vi "Send Text Using SMTP API 2013 NIVerified.vi"(2 "phone number 2":string, 3 "Carrier 2":enum16{"T-Mobile", "AT&T", "Verizon", "Sprint"}(ring), 4 "Body":string, 5 "Carrier 1":enum16{"T-Mobile", "AT&T", "Verizon", "Sprint"}(ring), 6 "Subject":string, 7 "phone number 1":string, 9 "Outgoing Mail Server (SMTP)":string="smtp.gmail.com", 10 "Password":string, 11 "Email":string) -> ()   [LabVIEW 2018]
uses:
  <vilib>/smtpClient/Set Message Text.vi
  <vilib>/smtpClient/LabVIEWSMTPClient.lvlib
panel:
  in  "TLS":bool=TRUE
  # "Overview\nThis example will allows you to use an SMTP server to send a SMS message to a cell phone.\nDescription\nWith the SMTP API you can send an email to your phone as a text message.  There are a lot of different servers you\n can use the default in this example is using GMAIL through the smtp.gmail.com server.  Most SMTP servers should \nwork, but the server and cell phone needs to be compatible to send and receive SMS messages.\nSteps to Implement or Execute Code\nOpen Send Text using SMTP API.vi\nFill in the SMTP server in the Outgoing Mail Server (SMTP), gmail is the default server\nFill out your email & Password\nSelect your Carrier and Type your Phone Number\nType the text you would like to send in the Body Control"
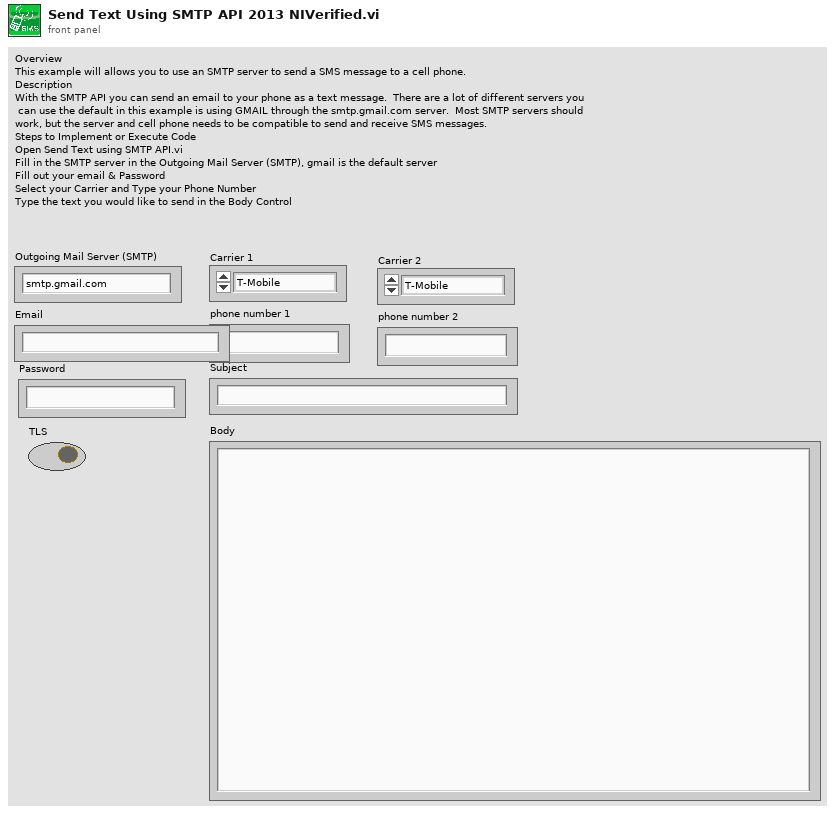
[diagram p1: front panel]
types:
  T1 = typedef "LabVIEWSMTPClient.lvlib/SmtpClientHandle.ctl" = refnum<k1>
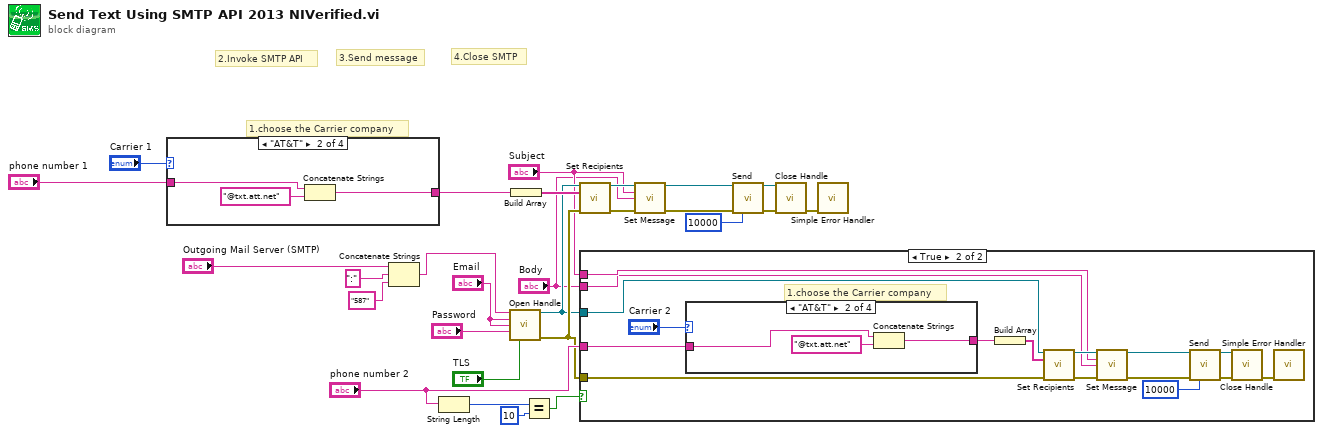
[diagram p0: block diagram]
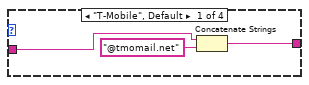
[diagram p3: hidden frame]
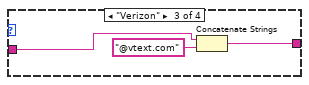
[diagram p4: hidden frame]
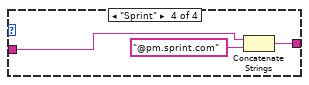
[diagram p5: hidden frame]
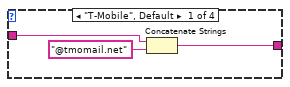
[diagram p6: hidden frame]
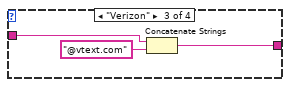
[diagram p7: hidden frame]
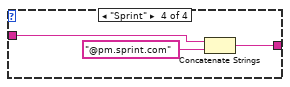
[diagram p8: hidden frame]
diagram:
  # "4.Close SMTP"
  # "3.Send message"
  # "2.Invoke SMTP API"
  # "1.choose the Carrier company"
  n1 = case shown="\"AT&T\"" "Carrier 1" {
    tunnel: "phone number 1" -> [w30 w32 w35 w38]
    tunnel: [w28 w33 w36 w39] -> w17
    frame "T-Mobile", Default {
      n2 = Concatenate Strings(w30, "@tmomail.net" ("string")) -> (w28:string)
    }
    frame "AT&T" {
      n3 = Concatenate Strings(w32, "@txt.att.net" ("string")) -> (w33:string)
    }
    frame "Verizon" {
      n4 = Concatenate Strings(w35, "@vtext.com" ("string")) -> (w36:string)
    }
    frame "Sprint" {
      n5 = Concatenate Strings(w38, "@pm.sprint.com") -> (w39:string)
    }
  }
  n6 = Concatenate Strings("Outgoing Mail Server (SMTP)", ":" ("string"), "587" ("Port")) -> (w12:string)
  n7 = String Length(string="phone number 2") -> (length=w7:i32)
  n8 = call <vilib>:"Open Handle.vi"("server address"=w12, "from"="Email", "username"="Email", "password"="Password", "use TLS (false)"="TLS") -> ("handle out"=w3:T1, "error out"=w4:errorcluster)  [unwired: 9 in]
  n9 = Build Array(w17) -> (w16:string[])
  n10 = Equal?(x=w7, y=10) -> (x = y?=w5:bool)
  n11 = call <vilib>:"Set Recipients.vi"("handle in"=w3, "to"=w16, "error in (no error)"=w4) -> ("handle out"=w23:T1, "error out"=w22:errorcluster)  [unwired: 11 in]
  n12 = case shown="True" w5 {
    tunnel: "phone number 2" -> [_ w55]
    tunnel: w4 -> [_ w43]
    tunnel: w3 -> [_ w42]
    tunnel: "Subject" -> [_ w41]
    tunnel: "Body" -> [_ w40]
    frame False {
    }
    frame True {
      # "1.choose the Carrier company"
      n13 = case shown="\"AT&T\"" "Carrier 2" {
        tunnel: w55 -> [w58 w60 w63 w66]
        tunnel: [w56 w61 w64 w67] -> w47
        frame "T-Mobile", Default {
          n14 = Concatenate Strings(w58, "@tmomail.net" ("string")) -> (w56:string)
        }
        frame "AT&T" {
          n15 = Concatenate Strings(w60, "@txt.att.net" ("string")) -> (w61:string)
        }
        frame "Verizon" {
          n16 = Concatenate Strings(w63, "@vtext.com" ("string")) -> (w64:string)
        }
        frame "Sprint" {
          n17 = Concatenate Strings(w66, "@pm.sprint.com") -> (w67:string)
        }
      }
      n18 = Build Array(w47) -> (w46:string[])
      n19 = call <vilib>:"Set Recipients.vi"("handle in"=w42, "to"=w46, "error in (no error)"=w43) -> ("handle out"=w53:T1, "error out"=w52:errorcluster)  [unwired: 11 in]
      n20 = call-poly <vilib>:"Set Message.vi"("handle in"=w53, "subject"=w41, "plain text message"=w40, "error in (no error)"=w52) -> ("handle out"=w51:T1, "error out"=w50:errorcluster)  [unwired: 10 in]
      n21 = call <vilib>:"Send.vi"("handle in"=w51, "error in (no error)"=w50, "timeout in ms (10000)"=10000) -> ("handle out"=w49:T1, "error out"=w48:errorcluster)  [unwired: 10 in, 1 out]
      n22 = call <vilib>:"Close Handle.vi"("handle in"=w49, "error in (no error)"=w48) -> ("error out"=w44:errorcluster)  [unwired: 12 in, 1 out]
      n23 = call <vilib>:"Simple Error Handler.vi"("error in (no error)"=w44) -> ()  [unwired: 4 in, 5 out]
    }
  }
  n24 = call-poly <vilib>:"Set Message.vi"("handle in"=w23, "subject"="Subject", "plain text message"="Body", "error in (no error)"=w22) -> ("handle out"=w21:T1, "error out"=w20:errorcluster)  [unwired: 10 in]
  n25 = call <vilib>:"Send.vi"("handle in"=w21, "error in (no error)"=w20, "timeout in ms (10000)"=10000) -> ("handle out"=w19:T1, "error out"=w18:errorcluster)  [unwired: 10 in, 1 out]
  n26 = call <vilib>:"Close Handle.vi"("handle in"=w19, "error in (no error)"=w18) -> ("error out"=w9:errorcluster)  [unwired: 12 in, 1 out]
  n27 = call <vilib>:"Simple Error Handler.vi"("error in (no error)"=w9) -> ()  [unwired: 4 in, 5 out]
